vi "Init Async State Vars.vi"(8 "Error in":errorcluster, 10 "Async Parameters":T6) -> (0 "Error out":errorcluster, 3 "Async State Vars":T1)   [LabVIEW 2017, in "Waveform-Processing-Custom-Device Engine.lvlib"]
uses:
  Waveform-Processing-Custom-Device Engine.lvlib
  Types/Async Parameters.ctl
  Types/Async FIFOs.ctl
  <vilib>/NI Veristand/Custom Device API/Waveform Data Reference.ctl
  Types/AsyncStateVariables.ctl
  <vilib>/NI Veristand/Custom Device Waveform API/Single Waveform Read (DBL)/Single Waveform Read (DBL).lvclass
  <vilib>/NI Veristand/Custom Device Waveform API/Single Waveform Write (DBL)/Single Waveform Write (DBL).lvclass
  Types/New Async FIFOs.ctl
  <vilib>/NI/NIVS Inline Async API/_Data Access Engine/Data Access Engine/Types/Write.DVR.ctl
  <vilib>/NI/NIVS Inline Async API/_Data Access Engine/Access Type Classes/Write/Write.lvclass
  <vilib>/NI/NIVS Inline Async API/_Data Access Engine/Data Access Engine/Types/Read.DVR.ctl
  <vilib>/NI/NIVS Inline Async API/_Data Access Engine/Access Type Classes/Read/Read.lvclass
  <vilib>/NI Veristand/Custom Device API/Custom Device API.lvlib
  <vilib>/NI/NIVS Inline Async API/_Data Access Engine/Data Access Engine/Data Access Engine.lvclass
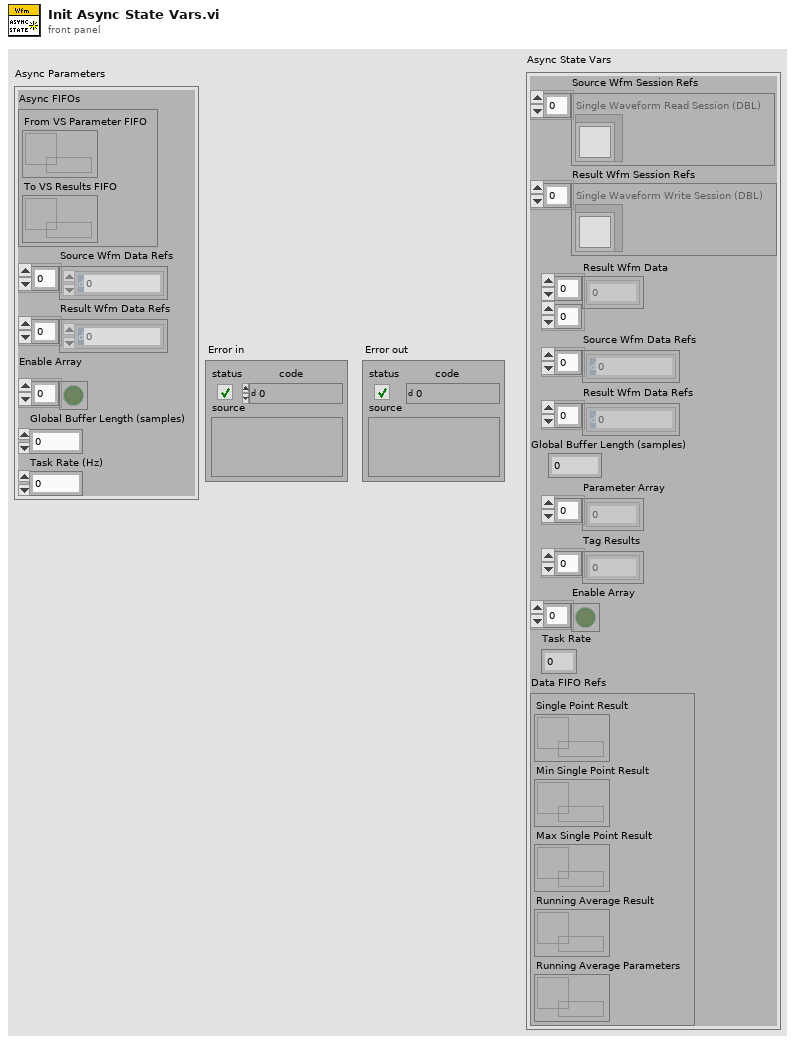
[diagram p1: front panel]
types:
  T1 = typedef "Waveform-Processing-Custom-Device Engine.lvlib/AsyncStateVariables.ctl" = cluster{"Source Wfm Session Refs":refnum<class "Single Waveform Read (DBL).lvclass">[], "Result Wfm Session Refs":refnum<class "Single Waveform Write (DBL).lvclass">[], "Result Wfm Data":dbl[][], "Source Wfm Data Refs":T2[], "Result Wfm Data Refs":T2[], "Global Buffer Length (samples)":dbl, "Parameter Array":dbl[], "Tag Results":dbl[], "Enable Array":bool[], "Task Rate":dbl, "Data FIFO Refs":T3}
  T2 = typedef "Custom Device API.lvlib/Waveform Data Reference.ctl" = i32
  T3 = typedef "Waveform-Processing-Custom-Device Engine.lvlib/New Async FIFOs.ctl" = cluster{"Single Point Result":T4, "Running Average Result":T4, "Running Average Parameters":T5, "Min Single Point Result":T4, "Max Single Point Result ":T4}
  T4 = typedef "Data Access Engine.lvlib/Data Access Engine.lvclass/Write.DVR.ctl" = refnum<data-value>
  T5 = typedef "Data Access Engine.lvlib/Data Access Engine.lvclass/Read.DVR.ctl" = refnum<data-value>
  T6 = typedef "Waveform-Processing-Custom-Device Engine.lvlib/Async Parameters.ctl" = cluster{"Async FIFOs":T7, "Source Wfm Data Refs":T2[], "Result Wfm Data Refs":T2[], "Enable Array":bool[], "Global Buffer Length (samples)":dbl, "Task Rate (Hz)":dbl}
  T7 = typedef "Waveform-Processing-Custom-Device Engine.lvlib/Async FIFOs.ctl" = cluster{"From VS Parameter FIFO":refnum<k33>, "To VS Results FIFO":refnum<k33>}
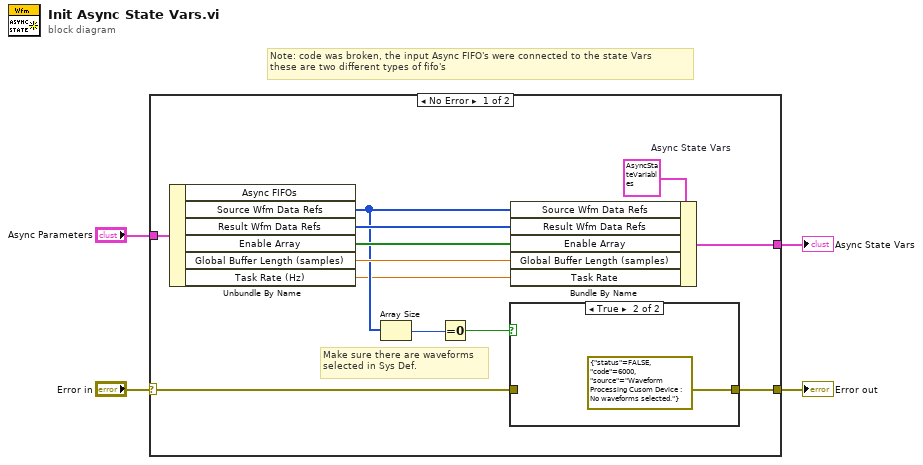
[diagram p0: block diagram]
diagram:
  # "Note: code was broken, the input Async FIFO's were connected to the state Vars \nthese are two different types of fifo's"
  n1 = case shown="No Error" "Error in" {
    selector: "Error in" -> [w7 w19]
    tunnel: [w6 w19] -> w3
    tunnel: "Async Parameters" -> [w16 _]
    tunnel: [w13 _] -> w1
    frame No Error {
      w15 = T1 {"Source Wfm Session Refs"=[], "Result Wfm Session Refs"=[], "Result Wfm Data"=[], "Source Wfm Data Refs"=[], "Result Wfm Data Refs"=[], "Global Buffer Length (samples)"=0.0, "Parameter Array"=[], "Tag Results"=[], "Enable Array"=[], "Task Rate"=0.0, "Data FIFO Refs"={"Single Point Result"=refnum, "Running Average Result"=refnum, "Running Average Parameters"=refnum, "Min Single Point Result"=refnum, "Max Single Point Result "=refnum}}  # Async State Vars
      # "Make sure there are waveforms\nselected in Sys Def."
      n2 = Unbundle By Name(w16) -> ("Source Wfm Data Refs"=w10:T2[], "Result Wfm Data Refs"=w14:T2[], "Enable Array"=w12:bool[], "Global Buffer Length (samples)"=w11:dbl, "Task Rate (Hz)"=w5:dbl)  [unwired: 1 out]
      n3 = Array Size(array=w10) -> (size(s)=w9:i32)
      n4 = Equal To 0?(x=w9) -> (x = 0?=w8:bool)
      n5 = case shown="True" w8 {
        tunnel: w7 -> [w17 _]
        tunnel: [w17 errorcluster {"status"=FALSE, "code"=6000, "source"="Waveform Processing Cusom Device : No waveforms selected."} ("error IO")] -> w6
        frame False {
        }
        frame True {
        }
      }
      n6 = Bundle By Name(cluster=w15, "Source Wfm Data Refs"=w10, "Result Wfm Data Refs"=w14, "Enable Array"=w12, "Global Buffer Length (samples)"=w11, "Task Rate"=w5) -> (w13:T1)
    }
    frame Error {
    }
  }
  "Error out" <- w3
  "Async State Vars" <- w1
